vi "RT Loop - TP Calc.vi"(11 "Message Queue":refnum<queue>) -> ()   [LabVIEW 2018]
doc: "This Control Loop VI performs control calculations of diverter line (DL) rotation."
uses:
  Support/Message Queue/Message Cluster.ctl
  Support/Message Queue/Message.ctl
  <vilib>/Platform/TimedLoop/XDataNode/timing_clust.ctl
  <vilib>/Platform/TimedLoop/XDataNode/nitl_modes.ctl
  <vilib>/Platform/TimedLoop/XDataNode/wakeup.ctl
  Controls/TP LCs.ctl
  <vilib>/Platform/TimedLoop/XDataNode/loadnilvce.vi
  Globals/Global - TP Channels.vi
  <vilib>/Platform/TimedLoop/XDataNode/XDataNode.xnode
  <vilib>/Platform/TimedLoop/XDataNode/XDNodeRunTimeDep.lvlib
  <vilib>/ptbypt/NI_PtbyPt.lvlib
  support/Message Queue/Message Queue.lvlib
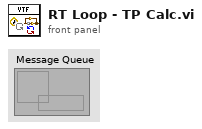
[diagram p1: front panel]
types:
  T1 = typedef "XDNodeRunTimeDep.lvlib/timing_clust.ctl" = cluster{"Expected End [f-1]":u64, "Actual End [f-1]":u64, "Finished Late? [f-1]":bool, "Expected End [i-1]":u64, "Actual End [i-1]":u64, "Finished Late? [i-1]":bool, "Expected Start [i]":u64, "Actual Start [i]":u64, "Expected Start [f]":u64, "Actual Start [f]":u64, "Source Name":string, "Structure Name":string, "Period":i64, "Deadline":i64, "Offset":i64, "Start":i64, "Priority":i32, "Timeout":i32, "Mode":T2, "Wakeup Reason":T3, "Error":errorcluster, "Source Type":string, "Secondary Source Type":string, "Global End Time":u64, "Global Start Time":u64, "Frame Duration":u64, "Iteration Duration":u64, "Assigned CPU":i32, "I/O Scan Engine Mode":u32}
  T2 = typedef "XDNodeRunTimeDep.lvlib/nitl_modes.ctl" = enum32{"No Change", "Process missed periods, maintain original phase", "Discard missed periods, maintain original phase", "Process missed periods, ignore original phase", "Discard missed periods, ignore original phase"}
  T3 = typedef "XDNodeRunTimeDep.lvlib/wakeup.ctl" = enum32{"Normal", "Aborted", "Asynchronous wakeup", "Timing source error", "Timed loop error", "Timeout"}
  T4 = typedef "TP LCs.ctl" = cluster{"TP LC1":dbl, "TP LC2":dbl, "TP LC3":dbl, "TP LC4":dbl, "TP Torque":dbl}
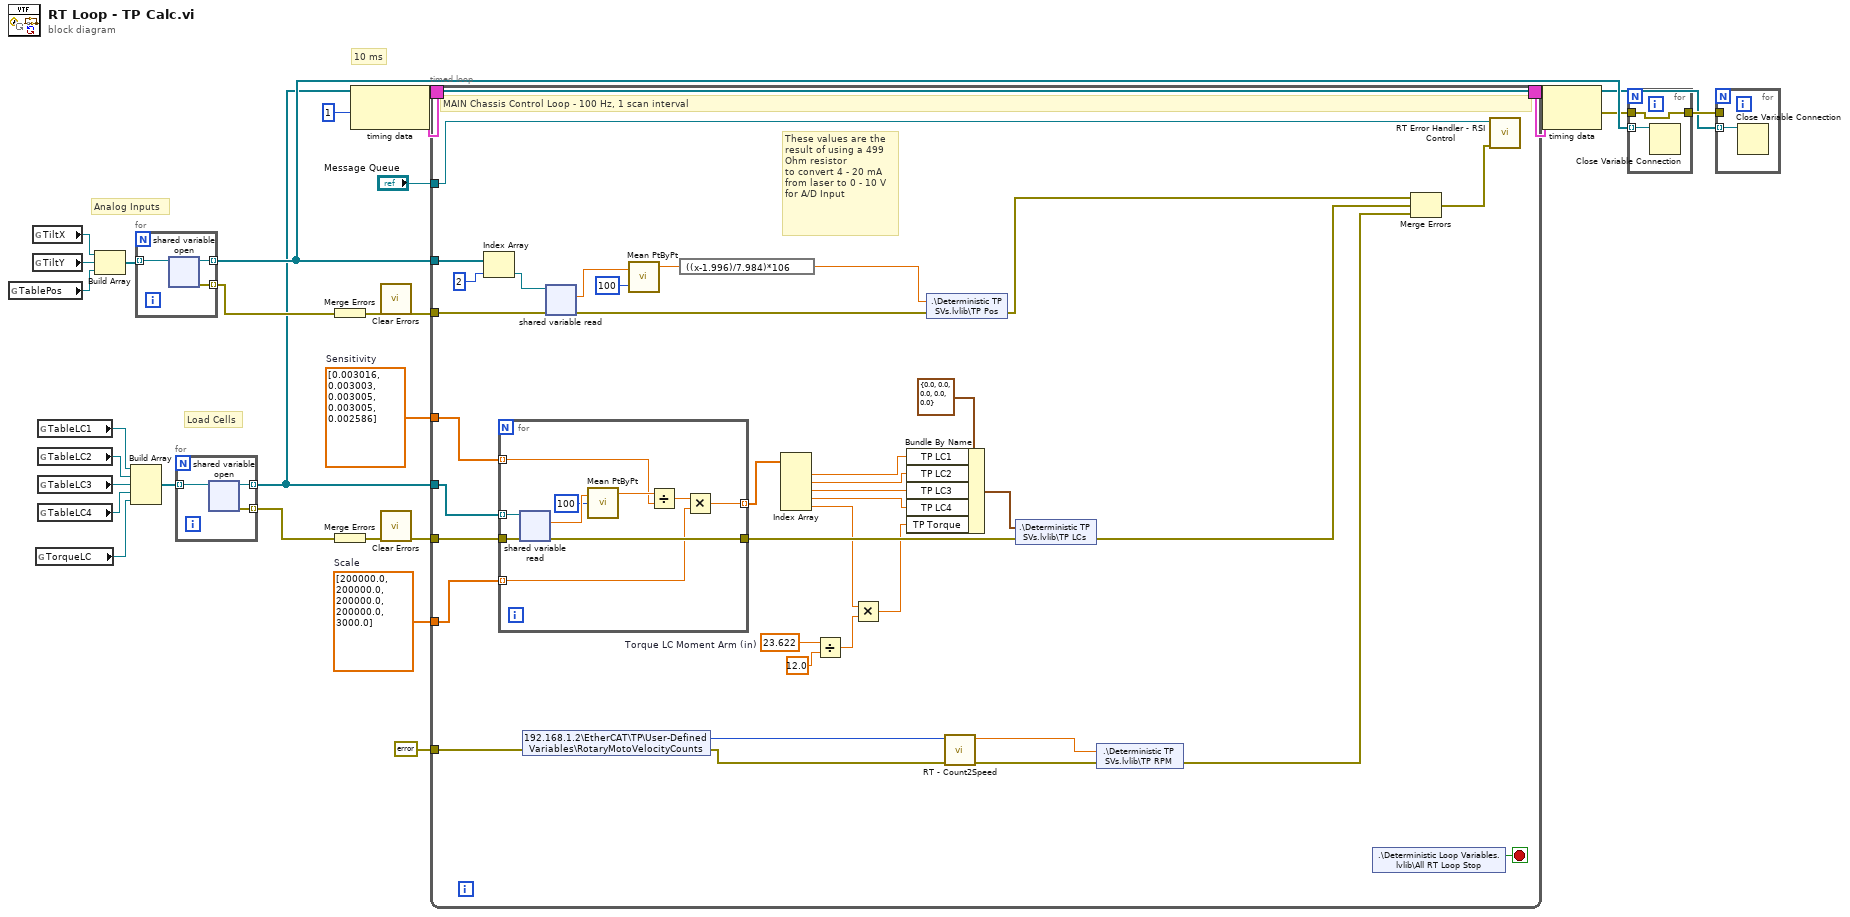
[diagram p0: block diagram]
diagram:
  w2 = dbl[] [200000.0, 200000.0, 200000.0, 200000.0, 3000.0]  # Scale
  w3 = dbl[] [0.003016, 0.003003, 0.003005, 0.003005, 0.002586]  # Sensitivity
  # "Load Cells"
  # "10 ms"
  # "Analog Inputs"
  n1 = global read "Global - TP Channels.vi" "TablePos"() -> (w15:refnum<k21>)
  n2 = global read "Global - TP Channels.vi" "TiltX"() -> (w17:refnum<k21>)
  n3 = global read "Global - TP Channels.vi" "TiltY"() -> (w16:refnum<k21>)
  n4 = global read "Global - TP Channels.vi" "TorqueLC"() -> (w10:refnum<k21>)
  n5 = global read "Global - TP Channels.vi" "TableLC1"() -> (w14:refnum<k21>)
  n6 = global read "Global - TP Channels.vi" "TableLC2"() -> (w13:refnum<k21>)
  n7 = global read "Global - TP Channels.vi" "TableLC3"() -> (w12:refnum<k21>)
  n8 = global read "Global - TP Channels.vi" "TableLC4"() -> (w11:refnum<k21>)
  n9 = Build Array(w17, w16, w15) -> (w18:refnum<k21>[])
  n10 = Build Array(w14, w13, w12, w11, w10) -> (w9:refnum<k21>[])
  n11 = for {
    tunnel: w18 -> [w30] mode=indexing
    tunnel: [w29] -> w22 mode=indexing
    tunnel: [w28] -> w19 mode=indexing
    n12 = shared-variable-open(w30) -> (w29:refnum<k21>, w28:errorcluster)  [unwired: 1 in]
  }
  n13 = for {
    tunnel: w9 -> [w33] mode=indexing
    tunnel: [w32] -> w4 mode=indexing
    tunnel: [w31] -> w7 mode=indexing
    n14 = shared-variable-open(w33) -> (w32:refnum<k21>, w31:errorcluster)  [unwired: 1 in]
  }
  n15 = Merge Errors(w19) -> (w20:errorcluster)
  n16 = Merge Errors(w7) -> (w8:errorcluster)
  n17 = node-c288(i64 1 ("Period")) -> (w27:T1)
  n18 = call <vilib>:"Clear Errors.vi"("error in (no error)"=w20) -> ("error out"=w23:errorcluster)  [unwired: 5 in, 1 out]
  n19 = call <vilib>:"Clear Errors.vi"("error in (no error)"=w8) -> ("error out"=w6:errorcluster)  [unwired: 5 in, 1 out]
  n20 = timed-loop {
    timing: w27 -> [_]
    timing-out: [_] -> w26
    tunnel: "Message Queue" -> [w68]
    tunnel: w23 -> [w69]
    tunnel: w22 -> [w67]
    tunnel: w6 -> [w58]
    tunnel: w4 -> [w59]
    tunnel: w3 -> [w46]
    tunnel: w2 -> [w45]
    tunnel: errorcluster {"status"=FALSE, "code"=0, "source"=""} ("error in (no error)") -> [w38]
    stop <- w70 stop-if-true
    w44 = 23.622  # Torque LC Moment Arm (in)
    # "These values are the result of using a 499 Ohm resistor\nto convert 4 - 20 mA from laser to 0 - 10 V for A/D Input"
    # "MAIN Chassis Control Loop - 100 Hz, 1 scan interval"
    n21 = Index Array(array=w67, index=2) -> (element=w65:refnum<k21>)
    n22 = for {
      tunnel: w59 -> [w80] mode=indexing
      tunnel: w58 -> [w79]
      tunnel: [w78] -> w53
      tunnel: w46 -> [w74] mode=indexing
      tunnel: w45 -> [w72] mode=indexing
      tunnel: [w71] -> w51 mode=indexing
      n23 = shared-variable-read(w80, w79) -> (w78:errorcluster, w77:dbl)  [unwired: 1 out]
      n24 = call <vilib>:"Mean PtByPt.vi"("x"=w77, "sample length"=100) -> ("mean"=w75:dbl)  [unwired: 2 in, 1 out]
      n25 = Divide(x=w75, y=w74) -> (x/y=w73:dbl)
      n26 = Multiply(x=w73, y=w72) -> (x*y=w71:dbl)
    }
    n27 = shared-variable "192.168.1.2\\EtherCAT\\TP\\User-Defined Variables\\RotaryMotoVelocityCounts"(error in=w38) -> (w39:i16, error out=w37:errorcluster)
    n28 = shared-variable-read(w65, w69) -> (w60:errorcluster, w64:dbl)  [unwired: 1 out]
    n29 = call <vilib>:"Mean PtByPt.vi"("x"=w64, "sample length"=100) -> ("mean"=w62:dbl)  [unwired: 2 in, 1 out]
    n30 = expression code="((x-1.996)/7.984)*106"(w62) -> (w61:dbl)
    n31 = Index Array(array=w51) -> (element #1=w50:dbl, element #2=w49:dbl, element #3=w48:dbl, element #4=w47:dbl, element #5=w41:dbl)  [unwired: 5 in]
    n32 = Divide(x=w44, y=12.0) -> (x/y=w42:dbl)
    n33 = Multiply(x=w41, y=w42) -> (x*y=w40:dbl)
    n34 = Bundle By Name(cluster=T4 {"TP LC1"=0.0, "TP LC2"=0.0, "TP LC3"=0.0, "TP LC4"=0.0, "TP Torque"=0.0} ("TP LCs"), "TP LC1"=w50, "TP LC2"=w49, "TP LC3"=w48, "TP LC4"=w47, "TP Torque"=w40) -> (w54:T4)
    n35 = shared-variable ".\\Deterministic TP SVs.lvlib\\TP Pos"(w61, error in=w60) -> (error out=w57:errorcluster)
    n36 = call "RT - Count2Speed.vi"("error in"=w37, "RotaryMotorVelocityCounts/Interval"=w39) -> ("error out"=w35:errorcluster, "Velocity (RPM)"=w36:dbl)  [unwired: 8 in]
    n37 = shared-variable ".\\Deterministic TP SVs.lvlib\\TP LCs"(w54, error in=w53) -> (error out=w52:errorcluster)
    n38 = shared-variable ".\\Deterministic TP SVs.lvlib\\TP RPM"(w36, error in=w35) -> (error out=w34:errorcluster)
    n39 = shared-variable ".\\Deterministic Loop Variables.lvlib\\All RT Loop Stop"() -> (w70:bool)  [unwired: 1 in, 1 out]
    n40 = Merge Errors(w57, w52, w34) -> (w56:errorcluster)
    n41 = call "RT Error Handler - RSI Control.vi"("error in (no error)"=w56, "Message Queue"=w68) -> ()  [unwired: 8 in, 2 out]
  }
  n42 = node-c288(w26) -> (w21:errorcluster)
  n43 = for {
    tunnel: w21 -> [w83]
    tunnel: w22 -> [w84] mode=indexing
    tunnel: [w83] -> w5
    n44 = Close Variable Connection(11:w84) -> ()  [unwired: 1 in, 1 out]
  }
  n45 = for {
    tunnel: w5 -> [_]
    tunnel: w4 -> [w85] mode=indexing
    n46 = Close Variable Connection(11:w85) -> ()  [unwired: 1 in, 1 out]
  }
